vi "ConfigSubPanel.vi"(11 "AllControls":T1) -> ()   [LabVIEW 2017]
uses:
  Ctrls/AllControls.ctl
  <vilib>/Utility/miscctls.llb/LVRowAndColumnTypeDef.ctl
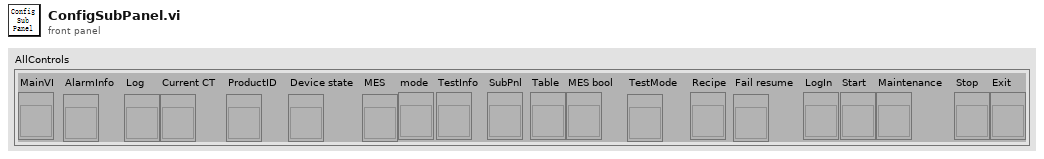
[diagram p1: front panel]
types:
  T1 = typedef "AllControls.ctl" = cluster{"MainVI":refnum<vi>, "AlarmInfo":refnum<vi>, "Log":refnum<vi>, "Current CT":refnum<vi>, "ProductID":refnum<vi>, "Device state":refnum<vi>, "MES":refnum<vi>, "mode":refnum<vi>, "TestInfo":refnum<vi>, "SubPnl":refnum<vi>, "Table":refnum<vi>, "MES bool":refnum<vi>, "TestMode":refnum<vi>, "Recipe":refnum<vi>, "Fail resume":refnum<vi>, "LogIn":refnum<vi>, "Start":refnum<vi>, "Maintenance":refnum<vi>, "Stop":refnum<vi>, "Exit":refnum<vi>}
  T2 = typedef "LVRowAndColumnTypeDef.ctl" = cluster{"Row":i32, "Column":i32}
  T3 = enum16{"Ini", "Standby", "Running", "Engineering"}
  T4 = typedef "Position Config.ctl" = cluster{"OrificeSize_12.7":i32, "OrificeSize_13":i32, "OrificeSize_30":i32, "OrificeSize_16":i32}
  T5 = typedef "HD Config.ctl" = cluster{" PC":cluster{"PC Address":u8[], "PC Port":i32}, "FCO":cluster{"COM":refnum<visa-resource-name>, "Baudrate":u32}, "DC Power ":cluster{"COM":refnum<visa-resource-name>, "Baudrate":u32}, "PW3336":cluster{"COM":refnum<visa-resource-name>, "Baudrate":u32}, "Lefoo":cluster{"COM":refnum<visa-resource-name>, "Baudrate":u32}, "AI Model":cluster{"COM":refnum<visa-resource-name>, "Baudrate":u32}, "DIPC":cluster{"COM":refnum<visa-resource-name>}, "RFID":cluster{"IP Address":string, "Port":u16, "Retry":u16}, "Motor":cluster{"COM":refnum<visa-resource-name>, "Baudrate":u32}, "Fail_resume_mode":bool, "GRR":bool}
  T6 = typedef "TesterInfo.ctl" = cluster{"Station Name":string, "Station Code":string, "ES NO.":string, "Tester ID":string, "PassMark Revision":string, "Rig ID":string, "Deamon_vision":string, "Project Name":string, "FFTesterPath":path, "Enable_User":bool, "Mode":enum16{"682"}, "MES":bool}
  T7 = enum32{"Bad", "Idle", "Run top level", "Running"}
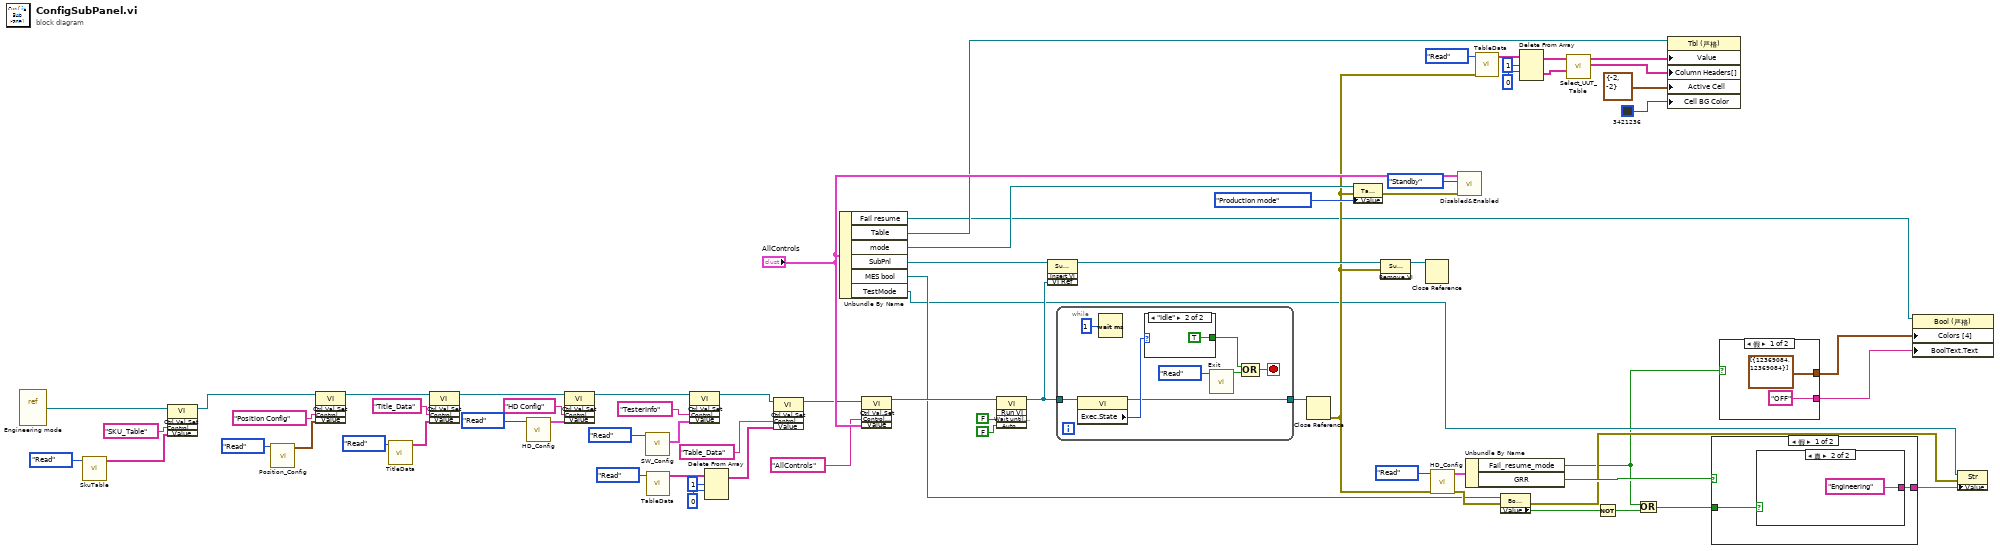
[diagram p0: block diagram]
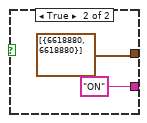
[diagram p2: hidden frame]
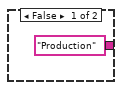
[diagram p3: hidden frame]
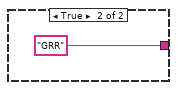
[diagram p4: hidden frame]
diagram:
  n1 = vi-ref "Engineering mode.vi"() -> (w3:refnum<vi>)
  n2 = call "SkuTable.vi"("Step"=enum16{"Initial", "Write", "Read"}."Read") -> ("Tabledata Out"=w1:string[][])  [unwired: 9 in, 1 out]
  n3 = invoke class="VI" method="Ctrl Val.Set"(reference=w3, "Control Name"="SKU_Table" ("控件名"), "Value"=w1) -> (reference out=w2:refnum<vi>)  [unwired: 2 in, 4 out]
  n4 = call "Position_Config.vi"("Step"=enum16{"Initial", "Write", "Read"}."Read") -> ("Position Config out"=w37:T4)  [unwired: 9 in, 1 out]
  n5 = invoke class="VI" method="Ctrl Val.Set"(reference=w2, "Control Name"="Position Config" ("控件名"), "Value"=w37) -> (reference out=w34:refnum<vi>)  [unwired: 2 in, 4 out]
  n6 = call "TitleData.vi"("Step"=enum16{"Initial", "Write", "Read"}."Read") -> ("Tabledata Out"=w32:string[][])  [unwired: 9 in, 1 out]
  n7 = invoke class="VI" method="Ctrl Val.Set"(reference=w34, "Control Name"="Title_Data" ("控件名"), "Value"=w32) -> (reference out=w33:refnum<vi>)  [unwired: 2 in, 4 out]
  n8 = call "HD_Config.vi"("Step"=enum16{"Initial", "Write", "Read"}."Read") -> ("HD Config out"=w61:T5)  [unwired: 9 in, 1 out]
  n9 = invoke class="VI" method="Ctrl Val.Set"(reference=w33, "Control Name"="HD Config" ("控件名"), "Value"=w61) -> (reference out=w57:refnum<vi>)  [unwired: 2 in, 4 out]
  n10 = call "SW_Config.vi"("Step"=enum16{"Initial", "Write", "Read"}."Read") -> ("SW Config out"=w46:T6)  [unwired: 9 in, 1 out]
  n11 = call "TableData.vi"("Step"=enum16{"Initial", "Write", "Read"}."Read") -> ("Tabledata Out"=w42:string[][])  [unwired: 9 in, 1 out]
  n12 = invoke class="VI" method="Ctrl Val.Set"(reference=w57, "Control Name"="TesterInfo" ("控件名"), "Value"=w46) -> (reference out=w49:refnum<vi>)  [unwired: 2 in, 4 out]
  n13 = Delete From Array(array=w42, length=1 ("长度"), index (row)=0 ("索引 (行)")) -> (array with subset deleted=w41:string[][])  [unwired: 1 in, 1 out]
  n14 = invoke class="VI" method="Ctrl Val.Set"(reference=w49, "Control Name"="Table_Data" ("控件名"), "Value"=w41) -> (reference out=w48:refnum<vi>)  [unwired: 2 in, 4 out]
  n15 = Unbundle By Name("AllControls") -> ("Fail resume"=w8:refnum<vi>, "Table"=w40:refnum<vi>, "mode"=w56:refnum<vi>, "SubPnl"=w65:refnum<vi>, "MES bool"=w22:refnum<vi>, "TestMode"=w21:refnum<vi>)
  n16 = invoke class="VI" method="Ctrl Val.Set"(reference=w48, "Control Name"="AllControls" ("控件名"), "Value"="AllControls") -> (reference out=w52:refnum<vi>)  [unwired: 2 in, 4 out]
  n17 = invoke class="VI" method="Run VI"(reference=w52, "Wait until done"=FALSE ("结束前等待"), "Auto Dispose Ref"=FALSE ("自动销毁引用")) -> (reference out=w67:refnum<vi>)  [unwired: 2 in, 4 out]
  n18 = invoke on="调用节点" class="SubPnl" method="Insert VI"(reference=w65, "VI Ref"=w67) -> (reference out=w63:refnum<vi>)  [unwired: 2 in, 3 out]
  n19 = while {
    tunnel: w67 -> [w70]
    tunnel: [w75] -> w62
    stop <- w74 stop-if-true
    n20 = property class="VI"(reference=w70) -> (reference out=w75:refnum<vi>, "Exec.State"=w77:T7)  [unwired: 1 in, 1 out]
    n21 = Wait (ms)(milliseconds to wait=u32 1 ("等待时间（毫秒）")) -> ()  [unwired: 1 out]
    n22 = case shown="\"Idle\"" w77 {
      tunnel: [_ TRUE] -> w76
      frame "Bad", Default {
      }
      frame "Idle" {
      }
    }
    n23 = call "Exit.vi"("Step"=enum16{"Initial", "Write", "Read"}."Read") -> ("Exit Out"=w72:bool)  [unwired: 9 in, 1 out]
    n24 = Compound Arithmetic op=OR ("复合运算")(w76, w72) -> (w74:bool)
  }
  n25 = Close Reference(reference=w62) -> (error out=w24:errorcluster)  [unwired: 1 in]
  n26 = property class="TabCtl (严格)"(reference=w56, error in=w24, "Value"=enum32{"Production mode", "Engineering mode"}."Production mode" ("值")) -> (error out=w53:errorcluster)  [unwired: 1 out]
  n27 = invoke on="调用节点" class="SubPnl" method="Remove VI"(reference=w63, error in=w24) -> (reference out=w64:refnum<vi>)  [unwired: 1 in, 2 out]
  n28 = Close Reference(reference=w64) -> ()  [unwired: 1 in, 1 out]
  n29 = call "HD_Config.vi"("error in (no error)"=w24, "Step"=enum16{"Initial", "Write", "Read"}."Read") -> ("error out"=w23:errorcluster, "HD Config out"=w25:T5)  [unwired: 8 in]
  n30 = call "Disabled&Enabled.vi"("error in (no error)"=w53, "Mode in"=T3."Standby", "AllControls In"="AllControls") -> ()  [unwired: 8 in, 1 out]
  n31 = Unbundle By Name(w25) -> ("Fail_resume_mode"=w9:bool, "GRR"=w31:bool)
  n32 = call "TableData.vi"("error in (no error)"=w24, "Step"=enum16{"Initial", "Write", "Read"}."Read") -> ("Tabledata Out"=w12:string[][])  [unwired: 8 in, 1 out]
  n33 = property class="Bool (严格)"(reference=w22, error in=w23) -> (error out=w20:errorcluster, "Value"=w29:bool)  [unwired: 1 out]
  n34 = Delete From Array(array=w12, length=1 ("长度"), index (row)=0 ("索引 (行)")) -> (deleted portion=w13:string[][], array with subset deleted=w15:string[][])  [unwired: 1 in]
  n35 = call "Select_UUT_Table.vi"("all Title"=w13, "all Table"=w15) -> ("Title"=w14:string[], "Table"=w7:string[][])  [unwired: 8 in]
  n36 = Not(x=w29) -> (.not. x?=w27:bool)
  n37 = Or(x=w9, y=w27) -> (x .or. y?=w28:bool)
  n38 = property class="Tbl (严格)"(reference=w40, "Value"=w7, "Column Headers[]"=w14, "Active Cell"=T2 {"Row"=-2, "Column"=-2} ("活动单元格:活动单元格"), "Cell BG Color"=u32 3421236) -> ()  [unwired: 1 in, 2 out]
  n39 = case shown="假" w31 {
    tunnel: w28 -> [w80 _]
    tunnel: [w79 "GRR"] -> w30
    frame False {
      n40 = case shown="真" w80 {
        tunnel: ["Production" "Engineering"] -> w79
        frame False {
        }
        frame True {
        }
      }
    }
    frame True {
    }
  }
  n41 = case shown="假" w9 {
    tunnel: [cluster{u32, u32}[] [{12369084, 12369084}] cluster{u32, u32}[] [{6618880, 6618880}]] -> w11
    tunnel: ["OFF" "ON"] -> w10
    frame False {
    }
    frame True {
    }
  }
  n42 = property on="属性节点" class="Bool (严格)"(reference=w8, "Colors [4]"=w11, "BoolText.Text"=w10) -> ()  [unwired: 1 in, 2 out]
  n43 = property class="Str"(reference=w21, error in=w20, "Value"=w30) -> ()  [unwired: 2 out]
